vi "Set Name.vi"(8 "error in (no error)":errorcluster, 10 "Key":string, 11 "Stack in":T1[](array[typedef])) -> (0 "error out":errorcluster, 3 "Stack out":T1[](array[typedef]))   [LabVIEW 2015, in "JSON.lvlib"]
uses:
  JSON.lvlib
  Context.ctl
  Object Context.ctl
  Name-Value Pair.ctl
  Value.ctl
  Value Type.ctl
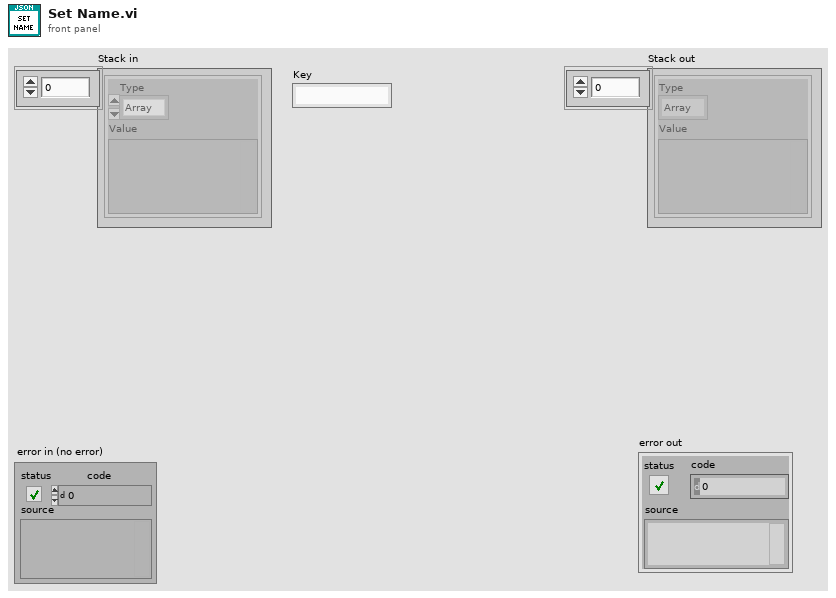
[diagram p1: front panel]
types:
  T1 = typedef "JSON.lvlib/Context.ctl" = cluster{"Type":enum16{"Array", "Object", "Root"}, "Value":variant}
  T2 = typedef "JSON.lvlib/Object Context.ctl" = cluster{"Object":T3[], "Key":string}
  T3 = typedef "JSON.lvlib/Name-Value Pair.ctl" = cluster{"Name":string, "Value":T4}
  T4 = typedef "JSON.lvlib/Value.ctl" = cluster{"Type":T5, "Value":variant}
  T5 = typedef "JSON.lvlib/Value Type.ctl" = enum16{"Object", "Array", "String", "Number", "Boolean", "Null"}
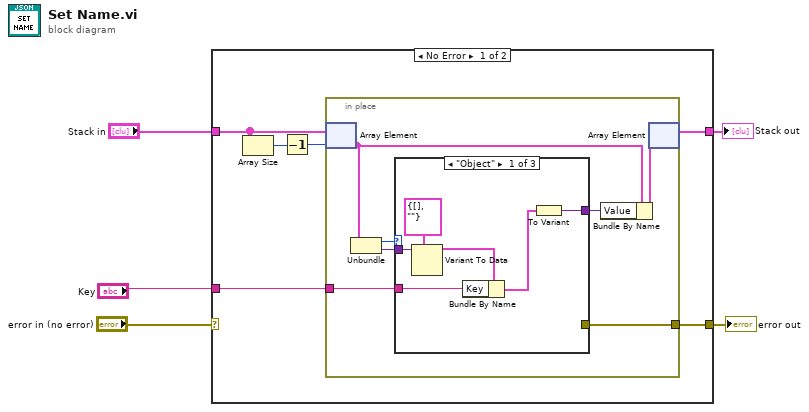
[diagram p0: block diagram]
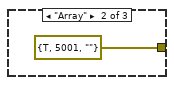
[diagram p2: hidden frame]
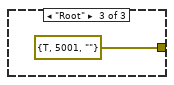
[diagram p3: hidden frame]
diagram:
  n1 = case shown="No Error" "error in (no error)" {
    selector: "error in (no error)" -> [_ w27]
    tunnel: "Stack in" -> [w9 w28]
    tunnel: [w8 w28] -> w4
    tunnel: "Key" -> [w7 _]
    tunnel: [w6 w27] -> w2
    frame No Error {
      n2 = Array Size(array=w9) -> (size(s)=w11:i32)
      n3 = Decrement(x=w11) -> (x-1=w10:i32)
      n4 = in-place {
        in-place-border: w7 -> [w16]
        in-place-border: [w12] -> w6
        n5 = in-place-array #1(w9, w10) -> (w15:T1)
        n6 = Unbundle(w15) -> ("Type"=w18:enum16{"Array", "Object", "Root"}, "Value"=w17:variant)
        n7 = case shown="\"Object\"" w18 {
          tunnel: w17 -> [w19 _ _]
          tunnel: w16 -> [w24 _ _]
          tunnel: [w22 _ _] -> w14
          tunnel: [_ errorcluster {"status"=TRUE, "code"=5001, "source"=""} ("error constant") errorcluster {"status"=TRUE, "code"=5001, "source"=""} ("error constant")] -> w12
          frame "Object" {
            n8 = Variant To Data(type=T2 {"Object"=[], "Key"=""} ("Table Context"), Variant=w19) -> (data=w20:T2)  [unwired: 1 in, 1 out]
            n9 = Bundle By Name(cluster=w20, "Key"=w24) -> (w23:T2)
            n10 = To Variant(anything=w23) -> (Variant=w22:variant)
          }
          frame "Array" {
          }
          frame "Root" {
          }
        }
        n11 = Bundle By Name(cluster=w15, "Value"=w14) -> (w13:T1)
        n12 = in-place-array #1(w13) -> (w8:T1[])  [unwired: 1 out]
      }
    }
    frame Error {
    }
  }
  "Stack out" <- w4
  "error out" <- w2
